vi "ex1-1.vi"() -> ()   [LabVIEW 2019]
panel:
  out "z":dbl
  out "y":dbl
  in  "a":dbl
  in  "x":dbl
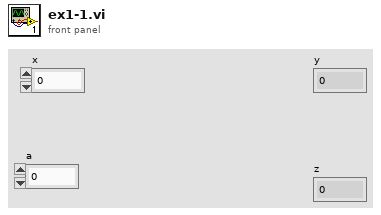
[diagram p1: front panel]
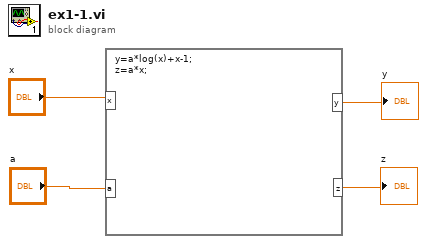
[diagram p0: block diagram]
diagram:
  n1 = formula code="y=a*log(x)+x-1;\nz=a*x;"("x"="x", "a"="a") -> ("y"=→"y":dbl, "z"=→"z":dbl)
